vi "动力和环境监控系统首页.vi"() -> ()   [LabVIEW 2016, in "环境动力监测库.lvlib"]
uses:
  <vilib>/Utility/miscctls.llb/LVRowAndColumnTypeDef.ctl
  <vilib>/Utility/config.llb/NI_LVConfig.lvlib
panel:
  in  "监测设备更新":bool
  in  "设备列表":i32(listbox)
  in  "add":bool
  out "设备当前时间:":timestamp format="%<%Y/%m/%d %H:%M:%S>T"
  out "当前传感器数量:":i32
  in  "设备":T1(ring)
  # "系统当前状态"
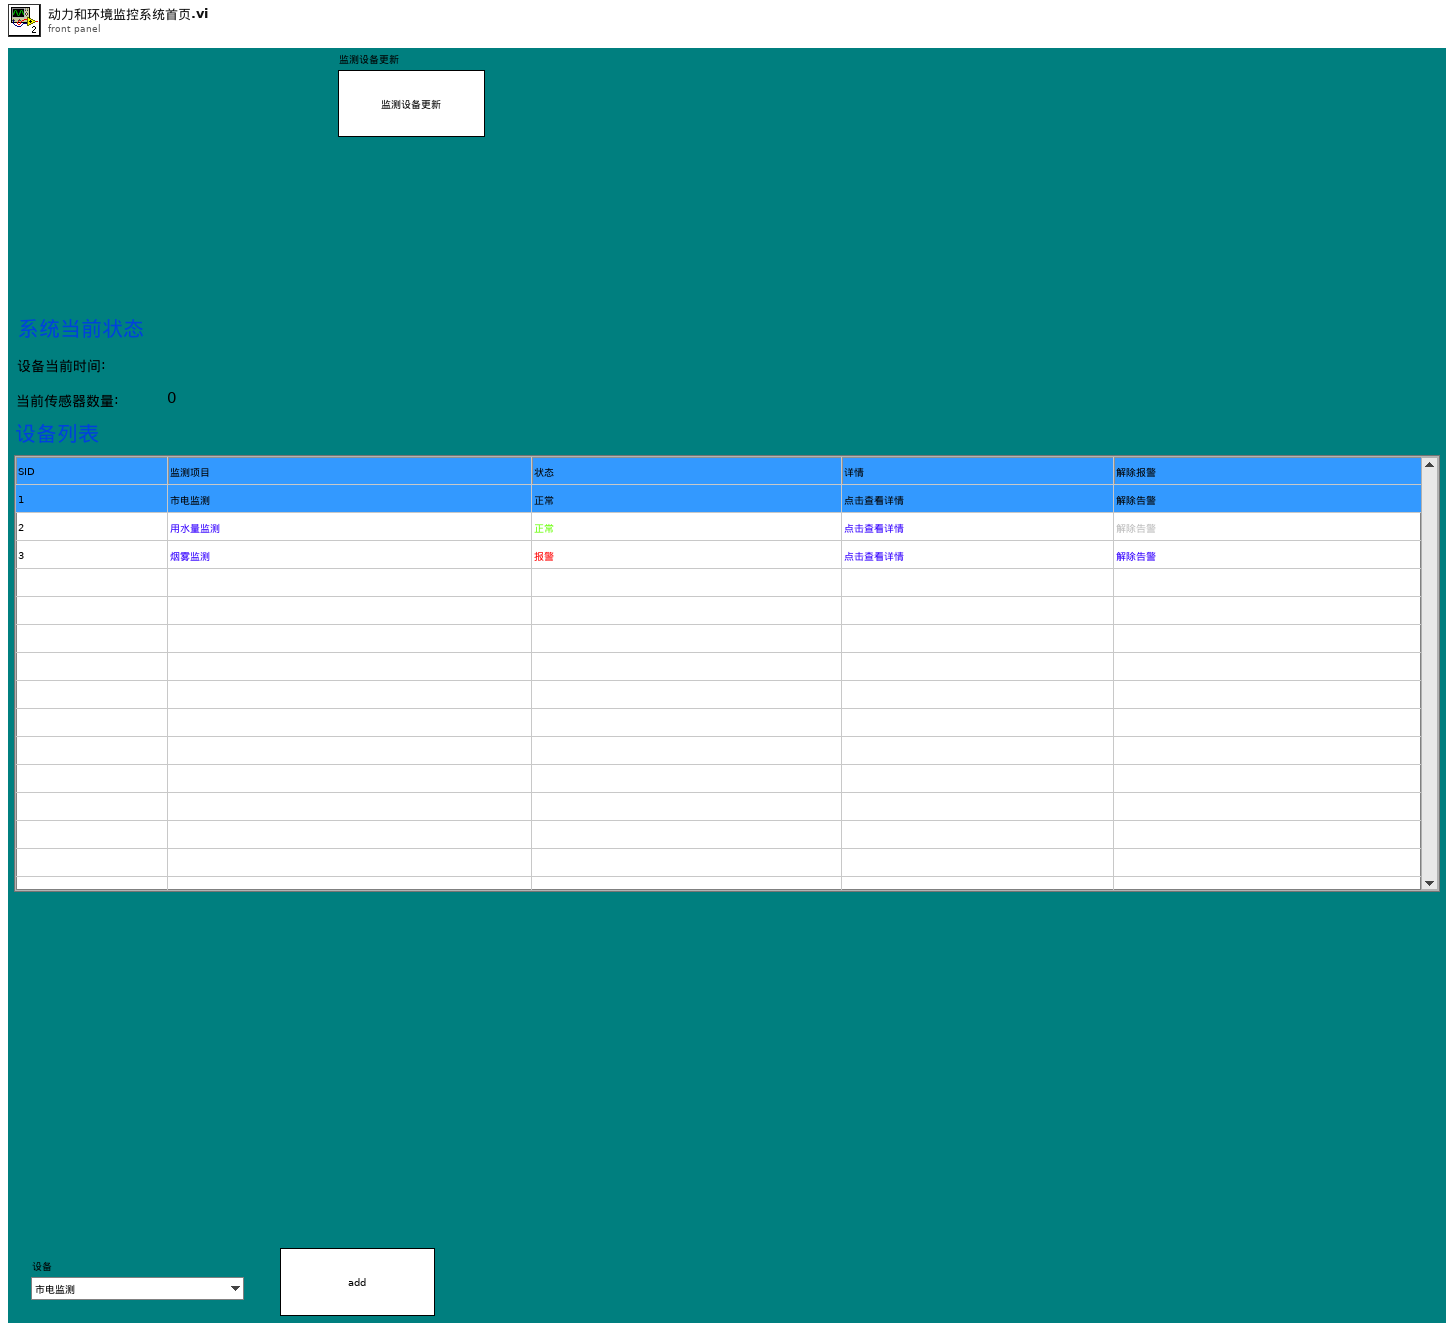
[diagram p1: front panel]
types:
  T1 = enum16{"市电监测", "UPS监测", "用水量监测", "空调监测", "烟雾监测", "温度湿度", "振动监测", "红外入侵监测", "漏水监测", "门禁开关监测", "视频监测"}
  T2 = typedef "NI_LVConfig.lvlib/Config Data RefNum.ctl" = refnum<k1>
  T3 = cluster{"市电监测":bool, "用水量监测":bool, "烟雾监测":bool, "温度湿度":bool, "振动监测":bool, "红外入侵监测":bool, "漏水监测":bool, "门禁开关监测":bool, "视频监测":bool, "UPS监测":bool, "空调监测":bool}
  T4 = enum32{"Invalid", "Standard", "Closed", "Hidden", "Minimized", "Maximized"}
  T5 = cluster{"漏水监测输出":bool, "门禁监测输出":bool, "温湿度监测输出":bool, "烟雾监测输出":bool, "空调监测输出":bool, "自动重合闸输出":bool}
  T6 = typedef "LVRowAndColumnTypeDef.ctl" = cluster{"Row":i32, "Column":i32}
  T7 = typedef "LVPoint32TypeDef.ctl" = cluster{"Horizontal":i32, "Vertical":i32}
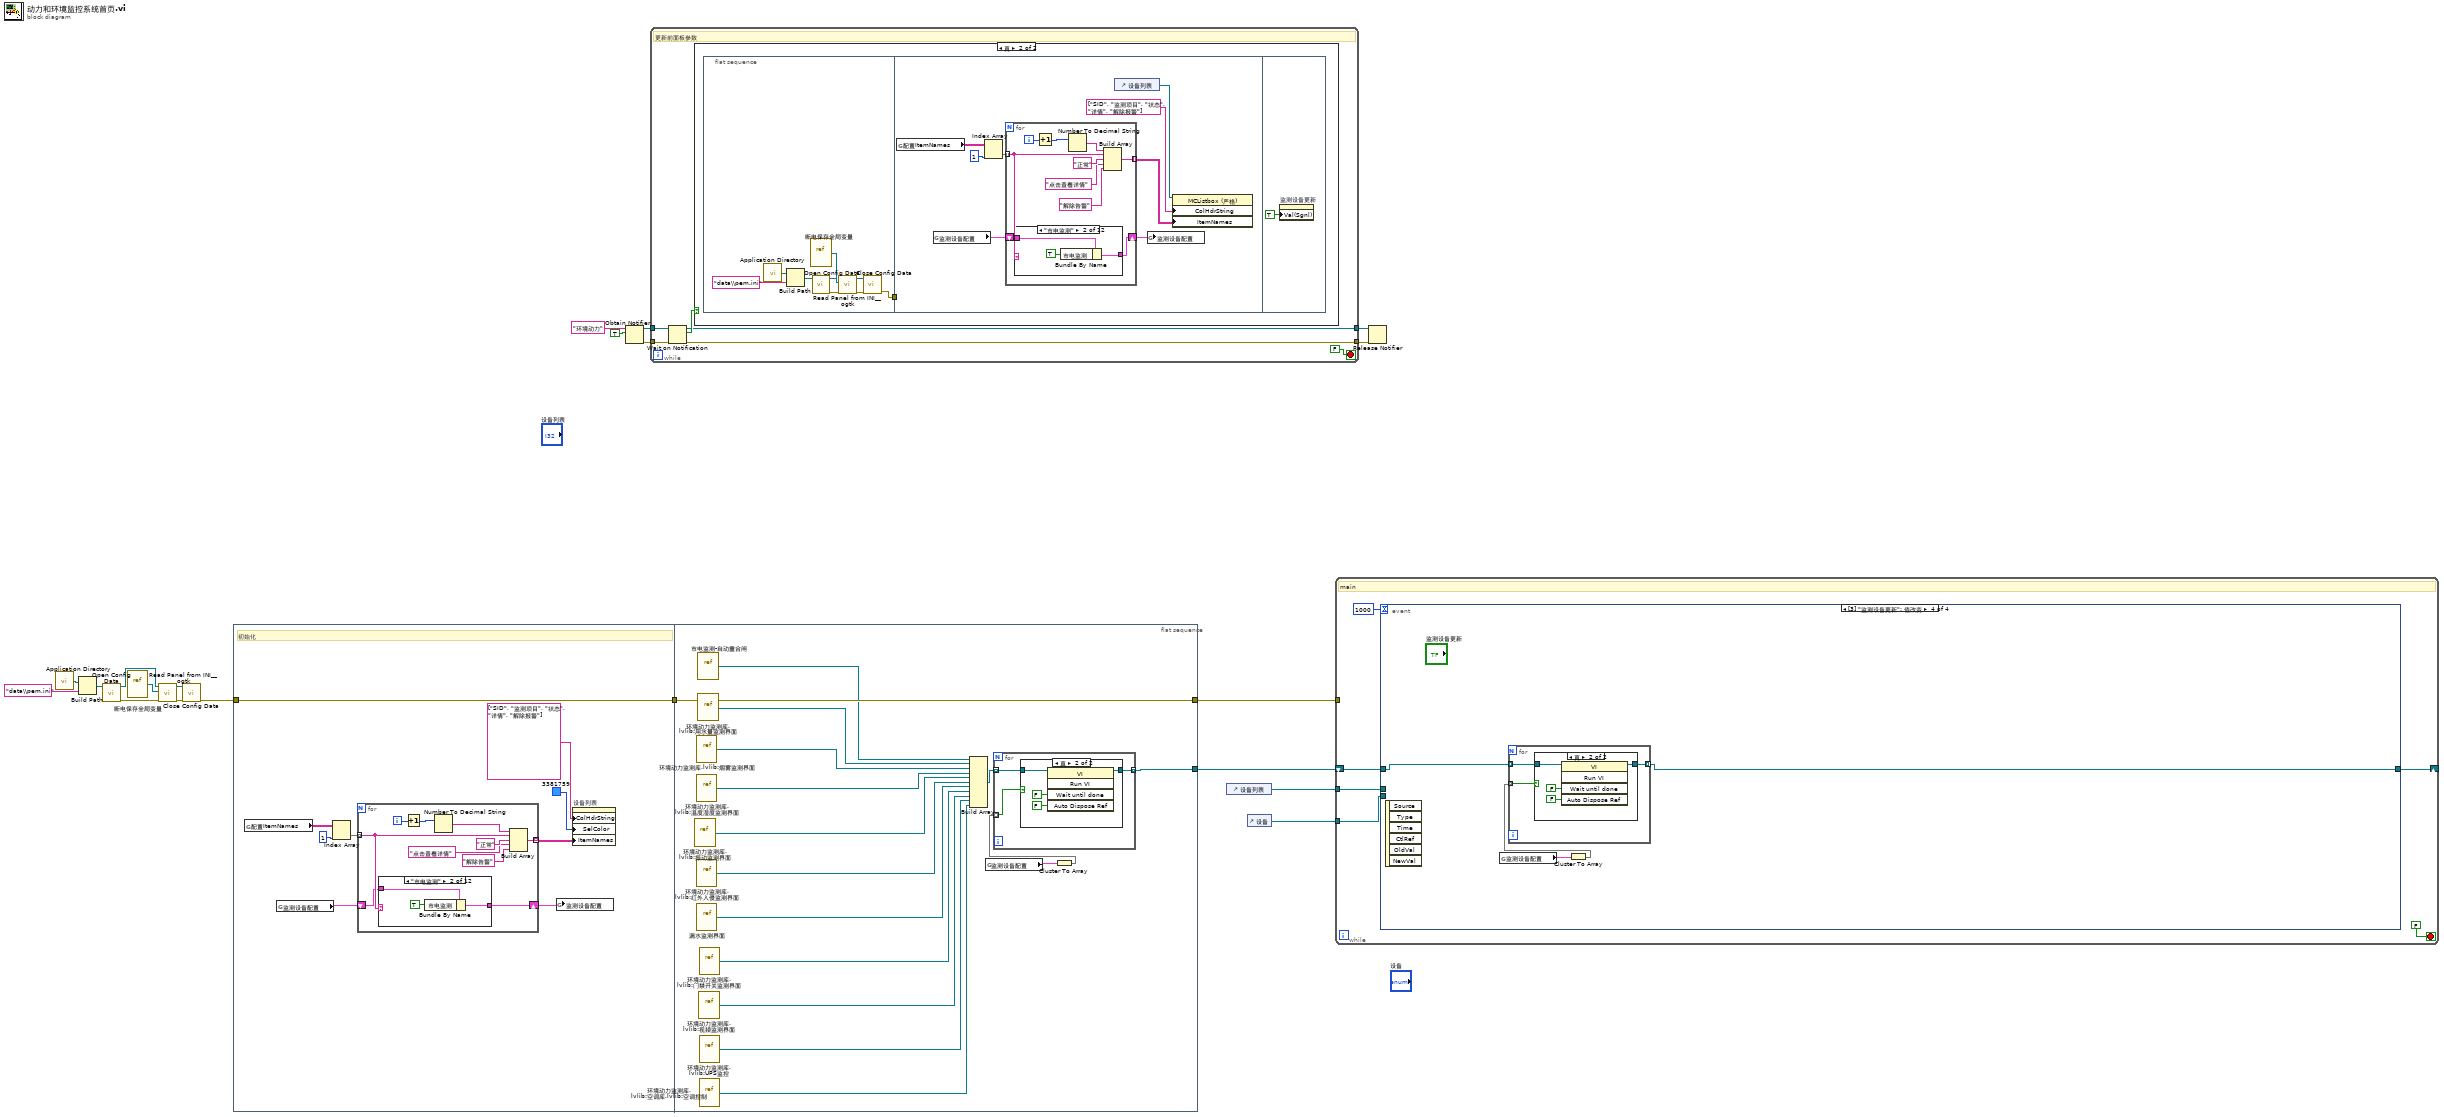
[diagram p0: block diagram]
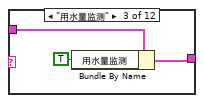
[diagram p4: hidden frame]
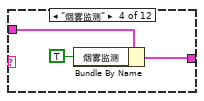
[diagram p5: hidden frame]
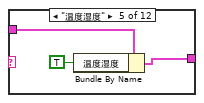
[diagram p6: hidden frame]
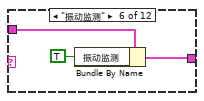
[diagram p7: hidden frame]
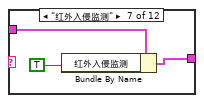
[diagram p8: hidden frame]
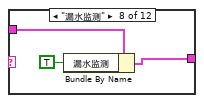
[diagram p9: hidden frame]
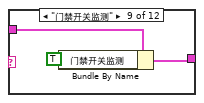
[diagram p10: hidden frame]
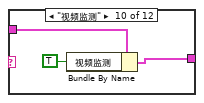
[diagram p11: hidden frame]
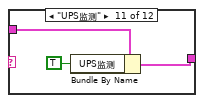
[diagram p12: hidden frame]
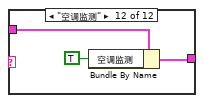
[diagram p13: hidden frame]
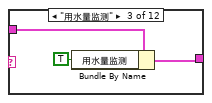
[diagram p15: hidden frame]
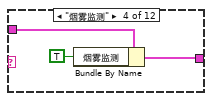
[diagram p16: hidden frame]
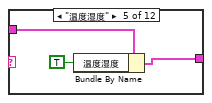
[diagram p17: hidden frame]
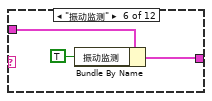
[diagram p18: hidden frame]
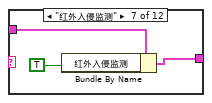
[diagram p19: hidden frame]
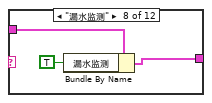
[diagram p20: hidden frame]
diagram:
  n1 = call <vilib>:"Application Directory.vi"() -> ("Application Directory"=w18:path)
  n2 = Build Path(base path=w18, name or relative path="data\\pem.ini" ("名称或相对路径")) -> (appended path=w16:path)
  n3 = call <vilib>:"Open Config Data.vi"("configuration file path"=w16) -> ("error out"=w12:errorcluster, "refnum"=w15:T2)  [unwired: 8 in, 1 out]
  n4 = vi-ref "断电保存全局变量.vi"() -> (w14:refnum<vi>)
  n5 = call <userlib>:"Read Panel from INI__ogtk.vi"("error in (no error)"=w12, "VI ref"=w14, "refnum"=w15) -> ("error out"=w11:errorcluster, "refnum out"=w13:T2)  [unwired: 7 in]
  n6 = call <vilib>:"Close Config Data.vi"("error in (no error)"=w11, "refnum"=w13) -> ("error out"=w10:errorcluster)  [unwired: 8 in, 1 out]
  n7 = flat-sequence {
    tunnel: w10 -> [w23]
    tunnel: [w23] -> w3
    tunnel: [w89] -> w1
    tunnel: w3 -> [w89]
    tunnel: [w74] -> w2
    frame #0 {
      # "初始化"
      n8 = global read "断电保存全局变量.vi" "配置ItemNames"() -> (w27:string[][])
      n9 = global read "内部交互全局变量.vi" "监测设备配置"() -> (w22:T3)
      n10 = Index Array(array=w27, index (col)=1 ("禁用的索引 (列)")) -> (element=w25:string[])  [unwired: 1 in]
      n11 = for {
        tunnel: w25 -> [w32] mode=indexing
        tunnel: [w33] -> w24 mode=indexing
        shift-right: [w30] -> w21
        shift-left: w22 -> [w31]
        i -> [w39]
        n12 = case shown="\"市电监测\"" w32 {
          tunnel: w31 -> [w40 w43 w45 w48 w51 w54 w57 w60 w63 w66 w69 w72]
          tunnel: [w40 w41 w44 w47 w50 w53 w56 w59 w62 w65 w68 w71] -> w30
          frame "假", Default {
          }
          frame "市电监测" {
            n13 = Bundle By Name(cluster=w43, "市电监测"=TRUE) -> (w41:T3)
          }
          frame "用水量监测" {
            n14 = Bundle By Name(cluster=w45, "用水量监测"=TRUE ("市电监测")) -> (w44:T3)
          }
          frame "烟雾监测" {
            n15 = Bundle By Name(cluster=w48, "烟雾监测"=TRUE ("市电监测")) -> (w47:T3)
          }
          frame "温度湿度" {
            n16 = Bundle By Name(cluster=w51, "温度湿度"=TRUE ("市电监测")) -> (w50:T3)
          }
          frame "振动监测" {
            n17 = Bundle By Name(cluster=w54, "振动监测"=TRUE ("市电监测")) -> (w53:T3)
          }
          frame "红外入侵监测" {
            n18 = Bundle By Name(cluster=w57, "红外入侵监测"=TRUE ("市电监测")) -> (w56:T3)
          }
          frame "漏水监测" {
            n19 = Bundle By Name(cluster=w60, "漏水监测"=TRUE ("市电监测")) -> (w59:T3)
          }
          frame "门禁开关监测" {
            n20 = Bundle By Name(cluster=w63, "门禁开关监测"=TRUE ("市电监测")) -> (w62:T3)
          }
          frame "视频监测" {
            n21 = Bundle By Name(cluster=w66, "视频监测"=TRUE ("市电监测")) -> (w65:T3)
          }
          frame "UPS监测" {
            n22 = Bundle By Name(cluster=w69, "UPS监测"=TRUE ("市电监测")) -> (w68:T3)
          }
          frame "空调监测" {
            n23 = Bundle By Name(cluster=w72, "空调监测"=TRUE ("市电监测")) -> (w71:T3)
          }
        }
        n24 = Increment(x=w39) -> (x+1=w38:i32)
        n25 = Number To Decimal String(number=w38) -> (decimal integer string=w37:string)  [unwired: 1 in]
        n26 = Build Array(w37, w32, "正常" ("元素"), "点击查看详情" ("元素"), "解除告警" ("元素")) -> (w33:string[])
      }
      n27 = global write "内部交互全局变量.vi" "监测设备配置"(w21) -> ()
      n28 = property on="设备列表" class="MCListbox (严格)"("ColHdrString"=string[] ["SID", "监测项目", "状态", "详情", "解除报警"] ("列首字符串[]"), "SelColor"=u32 3381759, "ItemNames"=w24) -> ()  [unwired: 2 in, 2 out]
    }
    frame #1 {
      n29 = vi-ref "环境动力监测库.lvlib:振动监测界面.vi"() -> (w80:refnum<vi>)
      n30 = vi-ref "环境动力监测库.lvlib:烟雾监测界面.vi"() -> (w78:refnum<vi>)
      n31 = vi-ref "环境动力监测库.lvlib:温度湿度监测界面.vi"() -> (w79:refnum<vi>)
      n32 = vi-ref "环境动力监测库.lvlib:红外入侵监测界面.vi"() -> (w81:refnum<vi>)
      n33 = vi-ref "漏水监测界面.vi"() -> (w82:refnum<vi>)
      n34 = vi-ref "市电监测-自动重合闸.vi"() -> (w76:refnum<vi>)
      n35 = vi-ref "环境动力监测库.lvlib:用水量监测界面.vi"() -> (w77:refnum<vi>)
      n36 = vi-ref "环境动力监测库.lvlib:视频监测界面.vi"() -> (w84:refnum<vi>)
      n37 = vi-ref "环境动力监测库.lvlib:门禁开关监测界面.vi"() -> (w83:refnum<vi>)
      n38 = vi-ref "环境动力监测库.lvlib:UPS监控.vi"() -> (w85:refnum<vi>)
      n39 = vi-ref "环境动力监测库.lvlib:空调库.lvlib:空调控制.vi"() -> (w86:refnum<vi>)
      n40 = Build Array(w76, w77, w78, w79, w80, w81, w82, w83, w84, w85, w86) -> (w75:refnum<vi>[])
      n41 = global read "内部交互全局变量.vi" "监测设备配置"() -> (w87:T3)
      n42 = Cluster To Array(cluster=w87) -> (array=w88:bool[])
      n43 = for {
        tunnel: w75 -> [w92] mode=indexing
        tunnel: [w91] -> w74 mode=indexing
        tunnel: w88 -> [w90] mode=indexing
        n44 = case shown="真" w90 {
          tunnel: w92 -> [w93 w95]
          tunnel: [w93 w94] -> w91
          frame False {
          }
          frame True {
            n45 = invoke class="VI" method="Run VI"(reference=w95, "Wait until done"=FALSE ("结束前等待"), "Auto Dispose Ref"=FALSE ("自动销毁引用")) -> (reference out=w94:refnum<vi>)  [unwired: 2 in, 4 out]
          }
        }
      }
    }
  }
  n46 = Obtain Notifier(name (unnamed)="环境动力" ("名称（未命名）"), notification data type=TRUE) -> (notifier out=w9:refnum<notifier>, error out=w8:errorcluster)  [unwired: 2 in, 1 out]
  n47 = while {
    tunnel: w9 -> [w103]
    tunnel: w8 -> [w102]
    tunnel: [w99] -> w5
    tunnel: [w98] -> w4
    stop <- FALSE stop-if-true
    # "更新前面板参数"
    n48 = Wait on Notification(notifier=w103, error in (no error)=w102) -> (notifier out=w99:refnum<notifier>, notification=w101:bool, error out=w98:errorcluster)  [unwired: 2 in, 1 out]
    n49 = case shown="真" w101 {
      frame False {
      }
      frame True {
        n50 = flat-sequence {
          tunnel: [w105] -> w104
          tunnel: w104 -> [_]
          frame #0 {
            n51 = call <vilib>:"Application Directory.vi"() -> ("Application Directory"=w106:path)
            n52 = Build Path(base path=w106, name or relative path="data\\pem.ini" ("名称或相对路径")) -> (appended path=w108:path)
            n53 = vi-ref "断电保存全局变量.vi"() -> (w110:refnum<vi>)
            n54 = call <vilib>:"Open Config Data.vi"("configuration file path"=w108) -> ("error out"=w112:errorcluster, "refnum"=w109:T2)  [unwired: 8 in, 1 out]
            n55 = call <userlib>:"Read Panel from INI__ogtk.vi"("error in (no error)"=w112, "VI ref"=w110, "refnum"=w109) -> ("error out"=w113:errorcluster, "refnum out"=w111:T2)  [unwired: 7 in]
            n56 = call <vilib>:"Close Config Data.vi"("error in (no error)"=w113, "refnum"=w111) -> ("error out"=w105:errorcluster)  [unwired: 8 in, 1 out]
          }
          frame #1 {
            n57 = global read "断电保存全局变量.vi" "配置ItemNames"() -> (w116:string[][])
            n58 = global read "内部交互全局变量.vi" "监测设备配置"() -> (w115:T3)
            n59 = Index Array(array=w116, index (col)=1 ("禁用的索引 (列)")) -> (element=w118:string[])  [unwired: 1 in]
            n60 = for {
              tunnel: w118 -> [w122] mode=indexing
              tunnel: [w125] -> w121 mode=indexing
              shift-right: [w123] -> w114
              shift-left: w115 -> [w124]
              i -> [w131]
              n61 = case shown="\"市电监测\"" w122 {
                tunnel: w124 -> [w132 w135 w137 w140 w143 w146 w149 w152 w155 w158 w161 w164]
                tunnel: [w132 w133 w136 w139 w142 w145 w148 w151 w154 w157 w160 w163] -> w123
                frame "假", Default {
                }
                frame "市电监测" {
                  n62 = Bundle By Name(cluster=w135, "市电监测"=TRUE) -> (w133:T3)
                }
                frame "用水量监测" {
                  n63 = Bundle By Name(cluster=w137, "用水量监测"=TRUE ("市电监测")) -> (w136:T3)
                }
                frame "烟雾监测" {
                  n64 = Bundle By Name(cluster=w140, "烟雾监测"=TRUE ("市电监测")) -> (w139:T3)
                }
                frame "温度湿度" {
                  n65 = Bundle By Name(cluster=w143, "温度湿度"=TRUE ("市电监测")) -> (w142:T3)
                }
                frame "振动监测" {
                  n66 = Bundle By Name(cluster=w146, "振动监测"=TRUE ("市电监测")) -> (w145:T3)
                }
                frame "红外入侵监测" {
                  n67 = Bundle By Name(cluster=w149, "红外入侵监测"=TRUE ("市电监测")) -> (w148:T3)
                }
                frame "漏水监测" {
                  n68 = Bundle By Name(cluster=w152, "漏水监测"=TRUE ("市电监测")) -> (w151:T3)
                }
                frame "门禁开关监测" {
                  n69 = Bundle By Name(cluster=w155, "门禁开关监测"=TRUE ("市电监测")) -> (w154:T3)
                }
                frame "视频监测" {
                  n70 = Bundle By Name(cluster=w158, "视频监测"=TRUE ("市电监测")) -> (w157:T3)
                }
                frame "UPS监测" {
                  n71 = Bundle By Name(cluster=w161, "UPS监测"=TRUE ("市电监测")) -> (w160:T3)
                }
                frame "空调监测" {
                  n72 = Bundle By Name(cluster=w164, "空调监测"=TRUE ("市电监测")) -> (w163:T3)
                }
              }
              n73 = Increment(x=w131) -> (x+1=w130:i32)
              n74 = Number To Decimal String(number=w130) -> (decimal integer string=w129:string)  [unwired: 1 in]
              n75 = Build Array(w129, w122, "正常" ("元素"), "点击查看详情" ("元素"), "解除告警" ("元素")) -> (w125:string[])
            }
            n76 = control-ref of="设备列表"() -> (w119:refnum<vi>)
            n77 = global write "内部交互全局变量.vi" "监测设备配置"(w114) -> ()
            n78 = property class="MCListbox (严格)"(reference=w119, "ColHdrString"=string[] ["SID", "监测项目", "状态", "详情", "解除报警"] ("列首字符串[]"), "ItemNames"=w121) -> ()  [unwired: 1 in, 2 out]
          }
          frame #2 {
            n79 = property on="监测设备更新" class="Bool (严格)"("Val(Sgnl)"=TRUE ("值(信号)")) -> ()  [unwired: 2 in, 2 out]
          }
        }
      }
    }
  }
  n80 = control-ref of="设备列表"() -> (w20:refnum<vi>)
  n81 = control-ref of="设备"() -> (w19:refnum<vi>)
  n82 = while {
    tunnel: w20 -> [w171]
    tunnel: w19 -> [w170]
    tunnel: w1 -> [_]
    shift-right: [w167] -> _
    shift-left: w2 -> [w168]
    stop <- FALSE stop-if-true
    # "main"
    n83 = event shown="[3] \"监测设备更新\": 值改变" {
      selector: _ -> [_ _ _ _]
      dyn-events: _ -> [_ _ _ _]
      timeout: 1000 -> [_ _ _ _]
      tunnel: w171 -> [_ w255 w262 _]
      tunnel: w170 -> [_ w254 _ _]
      tunnel: w168 -> [w173 w229 w256 w346]
      tunnel: [w173 w229 w256 w345] -> w167
      event Timeout {
        n84 = event-data() -> ()  [unwired: 1 in, 3 out]
        n85 = Get Date/Time In Seconds() -> (seconds since 1Jan1904=→"设备当前时间:":timestamp)
        n86 = property on="设备列表" class="MCListbox (严格)"() -> (error out=w175:errorcluster, "ItemNames"=w185:string[][])  [unwired: 2 in, 1 out]
        n87 = global read "内部交互全局变量.vi" "监测配置输出"() -> (w182:T5)
        n88 = Array Size(array=w185) -> (size(s)=w191:i32[])
        n89 = Index Array(array=w185, index (col) #1=1 ("禁用的索引 (列)"), index (col) #2=2 ("索引 (列)")) -> (element #1=w183:string[], element #2=w180:string[])  [unwired: 2 in]
        n90 = for {
          tunnel: w183 -> [w207] mode=indexing
          tunnel: w182 -> [w206]
          shift-right: [w202] -> w177
          shift-left: w180 -> [w204]
          tunnel: w175 -> [w198]
          tunnel: [w197] -> w174
          i -> [w195]
          w196 = T6 {"Row"=0, "Column"=0} ("活动单元格:活动单元格")
          n91 = case shown="\"市电监测\"" w207 {
            tunnel: w206 -> [_ w216 w218 w220 w222 w224 w226]
            tunnel: [TRUE ("烟雾监测输出") w215 w217 w219 w221 w223 w225] -> w205
            frame "假", Default {
            }
            frame "市电监测" {
              n92 = Unbundle By Name(w216) -> ("自动重合闸输出"=w215:bool)
            }
            frame "空调监测" {
              n93 = Unbundle By Name(w218) -> ("空调监测输出"=w217:bool)
            }
            frame "漏水监测" {
              n94 = Unbundle By Name(w220) -> ("漏水监测输出"=w219:bool)
            }
            frame "门禁开关监测" {
              n95 = Unbundle By Name(w222) -> ("门禁监测输出"=w221:bool)
            }
            frame "温度湿度" {
              n96 = Unbundle By Name(w224) -> ("温湿度监测输出"=w223:bool)
            }
            frame "烟雾监测" {
              n97 = Unbundle By Name(w226) -> ("烟雾监测输出"=w225:bool)
            }
          }
          n98 = case shown="假" w205 {
            tunnel: ["报警" "正常"] -> w203
            tunnel: [u32 16711680 u32 6618880] -> w199
            tunnel: [u32 3342591 ("颜色盒") u32 12369084] -> w192
            frame False {
            }
            frame True {
            }
          }
          n99 = Bundle By Name(cluster=w196, "Row"=w195, "Column"=2) -> (w200:T6)
          n100 = Bundle By Name(cluster=w196, "Row"=w195, "Column"=4) -> (w193:T6)
          n101 = property on="设备列表" class="MCListbox (严格)"(error in=w198, "ActiveCell"=w200, "CellFontColor"=w199, "ActiveCell"=w193, "CellFontColor"=w192) -> (error out=w197:errorcluster)  [unwired: 1 in, 1 out]
          n102 = Replace Array Subset(array=w204, new element=w203, index=w195) -> (w202:string[])
        }
        n103 = Index Array(array=w191) -> (element=w186:i32)  [unwired: 1 in]
        "当前传感器数量:" <- w186
        n104 = for {
          N: w186 -> [_]
          tunnel: [w227] -> w190 mode=indexing
          i -> [w228]
          n105 = Increment(x=w228) -> (x+1=w227:i32)
        }
        n106 = Number To Decimal String(number=w190) -> (decimal integer string=w189:string[])  [unwired: 1 in]
        n107 = Replace Array Subset(array=w185, new element=w189, index (col)=0 ("禁用的索引 (列)")) -> (w179:string[][])  [unwired: 1 in]
        n108 = Replace Array Subset(array=w179, new element=w177, index (col)=2 ("禁用的索引 (列)")) -> (w176:string[][])  [unwired: 1 in]
        n109 = property on="设备列表" class="MCListbox (严格)"(error in=w174, "ItemNames"=w176) -> ()  [unwired: 1 in, 2 out]
      }
      event "add": Value Change {
        w231 = u32 3342591 ("颜色盒")
        n110 = event-data() -> ()  [unwired: 1 in, 6 out]
        n111 = property class="MCListbox (严格)"(reference=w255) -> (reference out=w244:refnum<vi>, "ItemNames"=w248:string[][])  [unwired: 1 in, 1 out]
        n112 = property class="Enum (严格)"(reference=w254) -> ("RingText.Text"=w253:string)  [unwired: 1 in, 2 out]
        n113 = Array Size(array=w248) -> (size(s)=w247:i32[])
        n114 = Index Array(array=w247) -> (element=w236:i32)  [unwired: 1 in]
        n115 = Increment(x=w236) -> (x+1=w246:i32)
        n116 = Number To Decimal String(number=w246) -> (decimal integer string=w245:string)  [unwired: 1 in]
        n117 = Build Array(w245, w253, "正常" ("元素"), "点击查看详情" ("元素"), "解除告警" ("元素")) -> (w252:string[])
        n118 = Build Array (concatenate)(w248, w252) -> (w233:string[][])
        n119 = Bundle(w236, "Column"=1) -> (w232:cluster{i32, "Column":i32})  [unwired: 1 in]
        n120 = Bundle(w236, "Column"=2) -> (w241:cluster{i32, "Column":i32})  [unwired: 1 in]
        n121 = Bundle(w236, "Column"=3) -> (w238:cluster{i32, "Column":i32})  [unwired: 1 in]
        n122 = Bundle(w236, "Column"=4) -> (w235:cluster{i32, "Column":i32})  [unwired: 1 in]
        n123 = property class="MCListbox (严格)"(reference=w244, "ItemNames"=w233, "ActiveCell"=w232, "CellFontColor"=w231, "CellFontBold"=TRUE ("活动单元格:单元格字体:斜体"), "ActiveCell"=w241, "CellFontColor"=u32 61277 ("颜色盒"), "ActiveCell"=w238, "CellFontColor"=w231, "ActiveCell"=w235, "CellFontColor"=u32 12369084 ("颜色盒")) -> ()  [unwired: 1 in, 2 out]
      }
      event "设备列表": Mouse Down {
        n124 = event-data() -> ("CtlRef"=w268:refnum<vi>, "Coords"=w266:T7)  [unwired: 1 in, 6 out]
        n125 = property class="MCListbox (严格)"(reference=w262) -> (reference out=w258:refnum<vi>, "ItemNames"=w261:string[][])  [unwired: 1 in, 1 out]
        n126 = invoke class="MCListbox (严格)" method="Point To Row Column"(reference=w268, "Point"=w266) -> ("CellPosition"=w265:T6)  [unwired: 5 in, 6 out]
        n127 = Unbundle By Name(w265) -> ("Row"=w264:i32, "Column"=w267:i32)
        n128 = Array Size(array=w261) -> (size(s)=w260:i32[])
        n129 = Index Array(array=w260) -> (element=w259:i32)  [unwired: 1 in]
        n130 = In Range and Coerce(upper limit=w259, x=w264, lower limit=0 ("下限")) -> (In Range?=w257:bool)  [unwired: 1 out]
        n131 = case shown="真" w257 {
          tunnel: w267 -> [_ w278]
          tunnel: w264 -> [_ w277]
          tunnel: w265 -> [_ w275]
          tunnel: w258 -> [_ w272]
          tunnel: w256 -> [_ w269]
          frame False {
          }
          frame True {
            # "非列首字符串"
            n132 = property class="MCListbox (严格)"(reference=w272, "CellBG"=u32 16777216) -> (reference out=w273:refnum<vi>)  [unwired: 1 in, 1 out]
            n133 = property class="MCListbox (严格)"(reference=w273, "ActiveCell"=w275, "CellBG"=u32 16777216) -> (reference out=w276:refnum<vi>, "ItemNames"=w279:string[][], "CellFontColor"=w270:u32)  [unwired: 1 in, 1 out]
            n134 = case shown="3" w278 {
              tunnel: w279 -> [_ w295 w337]
              tunnel: w277 -> [_ w293 w335]
              tunnel: w276 -> [_ _ w336]
              tunnel: w270 -> [_ _ w334]
              tunnel: w269 -> [_ w291 _]
              frame 0, Default {
              }
              frame 3 {
                # "查看详情分支"
                n135 = Index Array(array=w295, index (row)=w293, index (col)=1 ("禁用的索引 (列)")) -> (element=w292:string)
                n136 = Index Array(array=w291) -> (element #1=w290:refnum<vi>, element #2=w289:refnum<vi>, element #3=w288:refnum<vi>, element #4=w287:refnum<vi>, element #5=w286:refnum<vi>, element #6=w285:refnum<vi>, element #7=w284:refnum<vi>, element #8=w283:refnum<vi>, element #9=w282:refnum<vi>, element #10=w281:refnum<vi>, element #11=w280:refnum<vi>)  [unwired: 11 in]
                n137 = case shown="\"空调监测\"" w292 {
                  selector: w292 -> [w296 _ _ _ _ _ _ _ _ _ _ _]
                  tunnel: w290 -> [_ w299 _ _ _ _ _ _ _ _ _ _]
                  tunnel: w289 -> [_ _ w302 _ _ _ _ _ _ _ _ _]
                  tunnel: w288 -> [_ _ _ w305 _ _ _ _ _ _ _ _]
                  tunnel: w287 -> [_ _ _ _ w308 _ _ _ _ _ _ _]
                  tunnel: w286 -> [_ _ _ _ _ w311 _ _ _ _ _ _]
                  tunnel: w285 -> [_ _ _ _ _ _ w314 _ _ _ _ _]
                  tunnel: w284 -> [_ _ _ _ _ _ _ w317 _ _ _ _]
                  tunnel: w283 -> [_ _ _ _ _ _ _ _ w320 _ _ _]
                  tunnel: w282 -> [_ _ _ _ _ _ _ _ _ w323 _ _]
                  tunnel: w281 -> [_ _ _ _ _ _ _ _ _ _ w326 _]
                  tunnel: w280 -> [_ _ _ _ _ _ _ _ _ _ _ w329]
                  frame "假", Default {
                    n138 = Concatenate Strings(w296, "详情" ("字符串")) -> (w298:string)
                    n139 = One Button Dialog(message=w298) -> ()  [unwired: 1 in, 1 out]
                  }
                  frame "市电监测" {
                    n140 = invoke class="VI" method="FP.Open"(reference=w299, "Activate"=TRUE ("激活？"), "State"=T4."Standard" ("状态")) -> ()  [unwired: 2 in, 5 out]
                  }
                  frame "用水量监测" {
                    n141 = invoke class="VI" method="FP.Open"(reference=w302, "Activate"=TRUE ("激活？"), "State"=T4."Standard" ("状态")) -> ()  [unwired: 2 in, 5 out]
                  }
                  frame "烟雾监测" {
                    n142 = invoke class="VI" method="FP.Open"(reference=w305, "Activate"=TRUE ("激活？"), "State"=T4."Standard" ("状态")) -> ()  [unwired: 2 in, 5 out]
                  }
                  frame "温度湿度" {
                    n143 = invoke class="VI" method="FP.Open"(reference=w308, "Activate"=TRUE ("激活？"), "State"=T4."Standard" ("状态")) -> ()  [unwired: 2 in, 5 out]
                  }
                  frame "振动监测" {
                    n144 = invoke class="VI" method="FP.Open"(reference=w311, "Activate"=TRUE ("激活？"), "State"=T4."Standard" ("状态")) -> ()  [unwired: 2 in, 5 out]
                  }
                  frame "红外入侵监测" {
                    n145 = invoke class="VI" method="FP.Open"(reference=w314, "Activate"=TRUE ("激活？"), "State"=T4."Standard" ("状态")) -> ()  [unwired: 2 in, 5 out]
                  }
                  frame "漏水监测" {
                    n146 = invoke class="VI" method="FP.Open"(reference=w317, "Activate"=TRUE ("激活？"), "State"=T4."Standard" ("状态")) -> ()  [unwired: 2 in, 5 out]
                  }
                  frame "门禁开关监测" {
                    n147 = invoke class="VI" method="FP.Open"(reference=w320, "Activate"=TRUE ("激活？"), "State"=T4."Standard" ("状态")) -> ()  [unwired: 2 in, 5 out]
                  }
                  frame "视频监测" {
                    n148 = invoke class="VI" method="FP.Open"(reference=w323, "Activate"=TRUE ("激活？"), "State"=T4."Standard" ("状态")) -> ()  [unwired: 2 in, 5 out]
                  }
                  frame "UPS监测" {
                    n149 = invoke class="VI" method="FP.Open"(reference=w326, "Activate"=TRUE ("激活？"), "State"=T4."Standard" ("状态")) -> ()  [unwired: 2 in, 5 out]
                  }
                  frame "空调监测" {
                    n150 = invoke class="VI" method="FP.Open"(reference=w329, "Activate"=TRUE ("激活？"), "State"=T4."Standard" ("状态")) -> ()  [unwired: 2 in, 5 out]
                  }
                }
              }
              frame 4 {
                # "解除报警"
                n151 = Equal?(x=w334, y=u32 3342591 ("颜色盒")) -> (x = y?=w333:bool)
                n152 = case shown="真" w333 {
                  tunnel: w337 -> [_ w342]
                  tunnel: w336 -> [_ _]
                  tunnel: w335 -> [_ w341]
                  frame False {
                  }
                  frame True {
                    n153 = Index Array(array=w342, index (row)=w341, index (col)=1 ("禁用的索引 (列)")) -> (element=w339:string)
                    n154 = Format Into String(format string="是否解除%s报警？" ("消息"), w339) -> (resulting string=w343:string)  [unwired: 2 in, 1 out]
                    n155 = Two Button Dialog(message=w343) -> (T button?=w338:bool)  [unwired: 2 in]
                    n156 = case shown="真" w338 {
                      frame False {
                      }
                      frame True {
                        # "触发解除报警事件"
                      }
                    }
                  }
                }
              }
            }
          }
        }
      }
      event "监测设备更新": Value Change {
        n157 = event-data() -> ()  [unwired: 1 in, 6 out]
        n158 = global read "内部交互全局变量.vi" "监测设备配置"() -> (w348:T3)
        n159 = Cluster To Array(cluster=w348) -> (array=w347:bool[])
        n160 = for {
          tunnel: w346 -> [w351] mode=indexing
          tunnel: [w350] -> w345 mode=indexing
          tunnel: w347 -> [w349] mode=indexing
          n161 = case shown="真" w349 {
            tunnel: w351 -> [w352 w354]
            tunnel: [w352 w353] -> w350
            frame False {
            }
            frame True {
              n162 = invoke class="VI" method="Run VI"(reference=w354, "Wait until done"=FALSE ("结束前等待"), "Auto Dispose Ref"=FALSE ("自动销毁引用")) -> (reference out=w353:refnum<vi>)  [unwired: 2 in, 4 out]
            }
          }
        }
      }
    }
  }
  n163 = Release Notifier(notifier=w5, error in (no error)=w4) -> ()  [unwired: 1 in, 3 out]
